vi "Call Action Dynamic.vi"(8 "error in (no error)":errorcluster, 11 "Auton Action Base in":refnum<class "Auton Action Base.lvclass">) -> (0 "error out":errorcluster, 3 "Auton Action Base out":refnum<class "Auton Action Base.lvclass">)   [LabVIEW 2016, in "Auton Mode Base.lvclass"]
uses:
  Auton Mode Base.lvclass
  Actions/Actions Base/Auton Action Base.lvclass
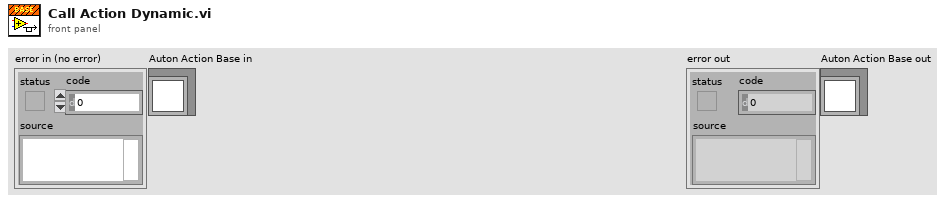
[diagram p1: front panel]
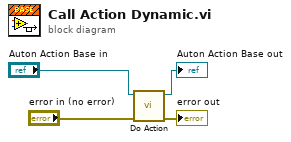
[diagram p0: block diagram]
diagram:
  n1 = call-dynamic "Do Action.vi"("error in (no error)"="error in (no error)", "Auton Action Base in"="Auton Action Base in") -> ("error out"=→"error out":errorcluster, "Auton Action Base out"=→"Auton Action Base out":refnum<class "Auton Action Base.lvclass">)  [unwired: 8 in]
